vi "Get Line Length From Line Number.vi"(11 "line number":enum8{"1 line", "2 lines"}(ring)) -> (3 "line length":u8)   [LabVIEW 2017, in "HD44780.lvclass"]
uses:
  HD44780.lvclass
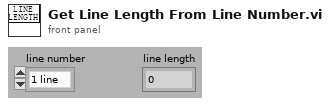
[diagram p1: front panel]
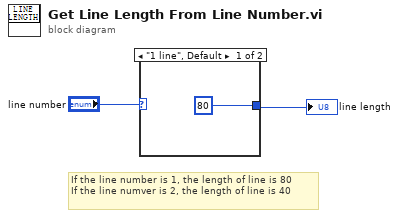
[diagram p0: block diagram]
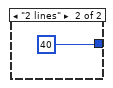
[diagram p2: hidden frame]
diagram:
  # "If the line number is 1, the length of line is 80\nIf the line numver is 2, the length of line is 40"
  n1 = case shown="\"1 line\", Default" "line number" {
    tunnel: [u8 80 u8 40] -> w2
    frame "1 line", Default {
    }
    frame "2 lines" {
    }
  }
  "line length" <- w2
